vi "Procura ponto médio.vi"(0 "Bounding Box":cluster{"x":sgl, "y":sgl}[](array[cluster])) -> (1 "Cluster":cluster{"x":sgl, "y":sgl}, 2 "X Médio":sgl, 3 "Y médio":sgl)   [LabVIEW 2020]
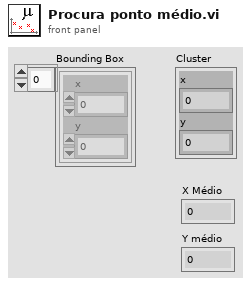
[diagram p1: front panel]
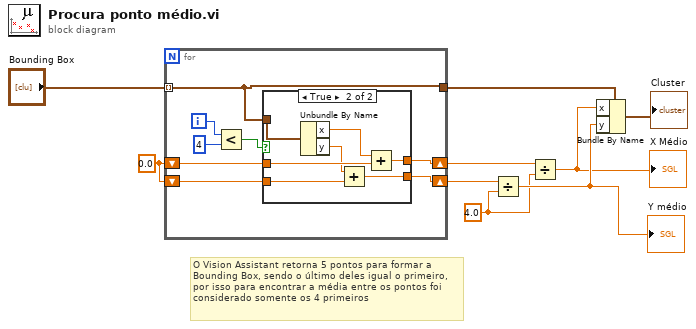
[diagram p0: block diagram]
diagram:
  w7 = sgl 0.0
  w3 = sgl 4.0 ("y")
  # "O Vision Assistant retorna 5 pontos para formar a Bounding Box, sendo o último deles igual o primeiro, por isso para encontrar a média entre os pontos foi considerado somente os 4 primeiros"
  n1 = for {
    tunnel: "Bounding Box" -> [w10] mode=indexing
    shift-right: [w17] -> w4
    shift-left: w7 -> [w16]
    shift-right: [w15] -> w2
    shift-left: w7 -> [w14]
    tunnel: [w10] -> w5
    i -> [w12]
    n2 = Less?(x=w12, y=4) -> (x < y?=w13:bool)
    n3 = case shown="True" w13 {
      tunnel: [w19 w26] -> w17
      tunnel: w16 -> [w19 w24]
      tunnel: [w18 w23] -> w15
      tunnel: w14 -> [w18 w22]
      tunnel: w10 -> [_ w20]
      frame False {
      }
      frame True {
        n4 = Unbundle By Name(w20) -> ("x"=w25:sgl, "y"=w21:sgl)
        n5 = Add(x=w21, y=w22) -> (x+y=w23:sgl)
        n6 = Add(x=w25, y=w24) -> (x+y=w26:sgl)
      }
    }
  }
  n7 = Divide(x=w2, y=w3) -> (x/y=w9:sgl)
  "Y médio" <- w9
  n8 = Divide(x=w4, y=w3) -> (x/y=w8:sgl)
  "X Médio" <- w8
  n9 = Bundle By Name(cluster=w5, "x"=w8, "y"=w9) -> (→"Cluster":cluster{"x":sgl, "y":sgl})
